vi "analyseImage.vi"(8 "error in (no error)":errorcluster, 10 "Array":T1(array[cluster]), 11 "FringeTesting in":refnum<class "FringeTesting.lvclass">) -> (0 "error out":errorcluster, 3 "FringeTesting out":refnum<class "FringeTesting.lvclass">)   [LabVIEW 2011, in "Tools.lvlib" / "Imaging.lvlib" / "FringeTesting.lvclass"]
uses:
  FringeTesting.lvclass
  Filing/FileNeologist/FileNeologist.lvclass
  ImageAnalyser.lvclass
  Filing/FileSystem/FileSystem.lvclass
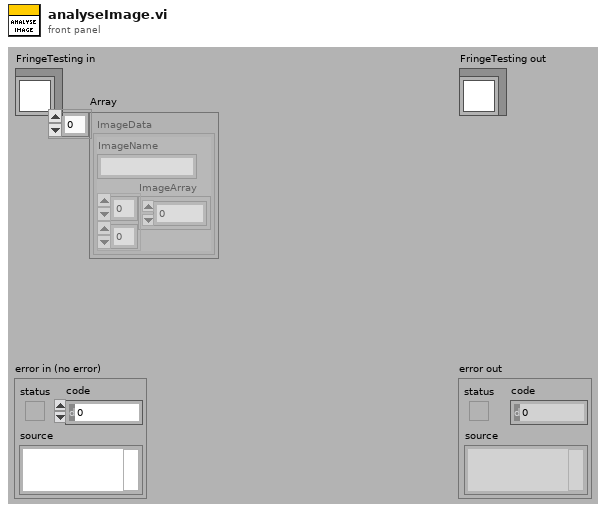
[diagram p1: front panel]
types:
  T1 = cluster{"ImageName":string, "ImageArray":sgl[][]}[]
  T2 = cluster{"Name":string, "Results":dbl[], "AnalysisType":string}
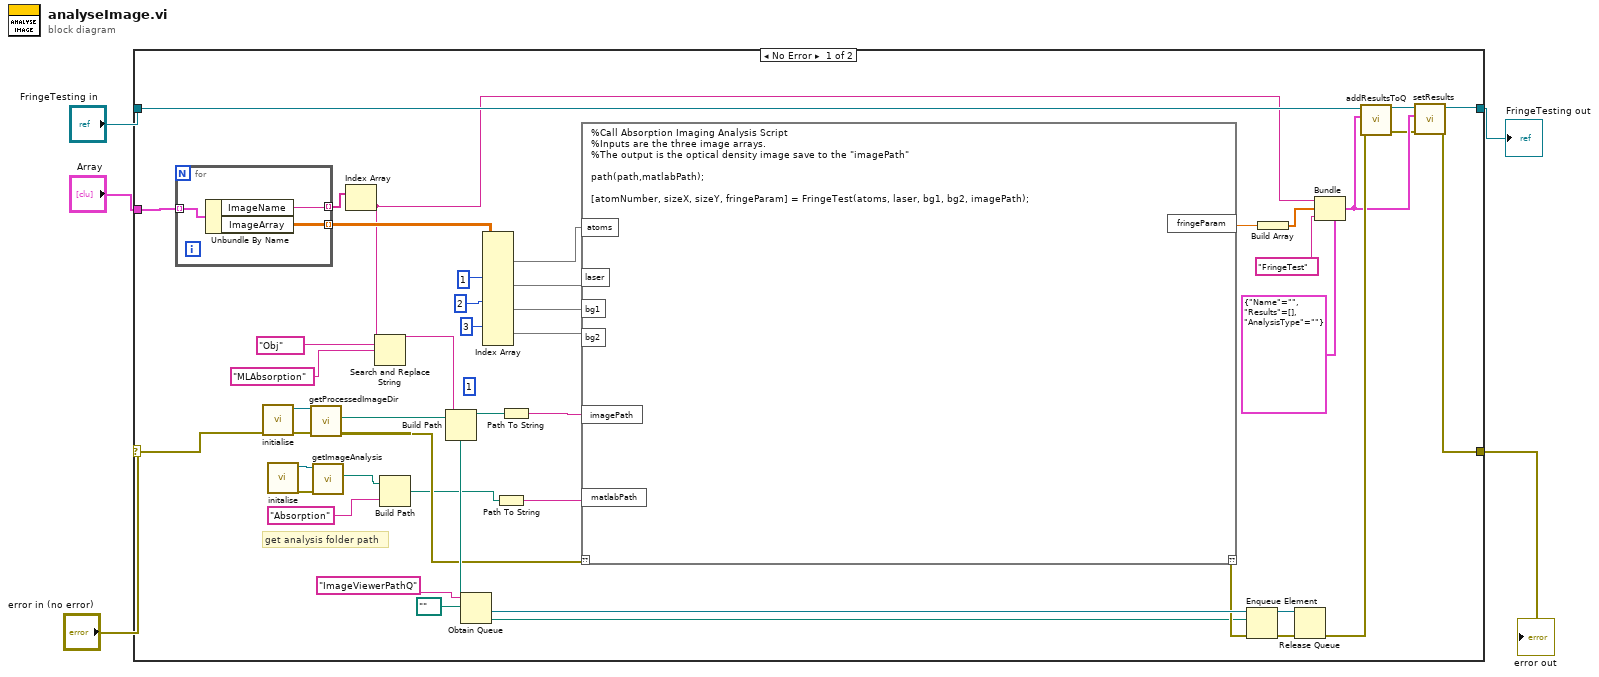
[diagram p0: block diagram]
diagram:
  n1 = case shown="No Error" "error in (no error)" {
    selector: "error in (no error)" -> [w21 w54]
    tunnel: [w9 w54] -> w2
    tunnel: [w12 w53] -> w1
    tunnel: "FringeTesting in" -> [w48 w53]
    tunnel: "Array" -> [w47 _]
    frame No Error {
      (unwired) 1
      # "get analysis folder path"
      n2 = for {
        tunnel: w47 -> [w52] mode=indexing
        tunnel: [w51] -> w46 mode=indexing
        tunnel: [w50] -> w42 mode=indexing
        n3 = Unbundle By Name(w52) -> ("ImageName"=w50:string, "ImageArray"=w51:sgl[][])
      }
      n4 = call "initialise.vi"("error in (no error)"=w21) -> ("error out"=w38:errorcluster, "FileNeologist out"=w39:refnum<class "FileNeologist.lvclass">)  [unwired: 9 in]
      n5 = call "initalise.vi"() -> ("error out"=w17:errorcluster, "FileSystem out"=w18:refnum<class "FileSystem.lvclass">)  [unwired: 10 in]
      n6 = call-dynamic "getProcessedImageDir.vi"("error in (no error)"=w38, "FileNeologist in"=w39) -> ("error out"=w20:errorcluster, "Path"=w37:path)  [unwired: 7 in, 1 out]
      n7 = call "getImageAnalysis.vi"("error in (no error)"=w17, "FileSystem in"=w18) -> ("ImageAnalysis"=w16:path)  [unwired: 7 in, 2 out]
      n8 = Index Array(array=w42) -> (element=w24:string)  [unwired: 1 in]
      n9 = Search and Replace String(input string=w24, search string="Obj", replace string="MLAbsorption") -> (result string=w36:string)  [unwired: 5 in, 3 out]
      n10 = Build Path(base path=w16, name or relative path="Absorption") -> (appended path=w14:path)
      n11 = Build Path(base path=w37, name or relative path=w36) -> (appended path=w27:path)
      n12 = Obtain Queue(name (unnamed)="ImageViewerPathQ", element data type=path "") -> (queue out=w33:refnum<queue>)  [unwired: 3 in, 2 out]
      n13 = Index Array(array=w46, index (dim 0) #2=1, index (dim 0) #3=2, index (dim 0) #4=3) -> (element #1=w6:sgl[][], element #2=w44:sgl[][], element #3=w43:sgl[][], element #4=w7:sgl[][])  [unwired: 9 in]
      n14 = Path To String(path=w14) -> (string=w19:string)
      n15 = Path To String(path=w27) -> (string=w30:string)
      n16 = script code="%Call Absorption Imaging Analysis Script \n%Inputs are the three image arrays.\n%The output is the optical density image save to the \"imagePath\"\n\npath(path,matlabPath);\n\n[atomNumber, sizeX, sizeY, fringeParam] = FringeTest(atoms, laser, bg1, bg2, imagePath);"("??"=w20, "bg1"=w43, "laser"=w44, "atoms"=w6, "imagePath"=w30, "matlabPath"=w19, "bg2"=w7) -> ("??"=w28:errorcluster, "fringeParam"=w29:dbl)
      n17 = Enqueue Element(queue=w33, element=w27, error in (no error)=w28) -> (queue out=w32:refnum<queue>, error out=w31:errorcluster)  [unwired: 1 in, 1 out]
      n18 = Build Array(w29) -> (w25:dbl[])
      n19 = Release Queue(queue=w32, error in (no error)=w31) -> (error out=w26:errorcluster)  [unwired: 1 in, 2 out]
      n20 = Bundle(cluster=T2 {"Name"="", "Results"=[], "AnalysisType"=""} ("output cluster"), "Name"=w24, "Results"=w25, "AnalysisType"="FringeTest") -> (w11:T2)
      n21 = call "addResultsToQ.vi"("error in (no error)"=w26, "Results"=w11, "ImageAnalyser in"=w48) -> ("error out"=w10:errorcluster, "ImageAnalyser out"=w13:refnum<class "FringeTesting.lvclass">)  [unwired: 7 in]
      n22 = call "setResults.vi"("error in (no error)"=w10, "results"=w11, "ImageAnalyser in"=w13) -> ("error out"=w9:errorcluster, "ImageAnalyser out"=w12:refnum<class "FringeTesting.lvclass">)  [unwired: 7 in]
    }
    frame Error {
    }
  }
  "error out" <- w2
  "FringeTesting out" <- w1
